vi "Read Firmware and Build Version.vi"(0 "Session Handle in":T1, 11 "error in (no error)":errorcluster) -> (4 "Session Handle out":T1, 6 "Build Date":string, 8 "Firmware Version":string, 15 "error out":errorcluster)   [LabVIEW 2015, in "PAS.lvclass"]
uses:
  PAS.lvclass
  Typedefs/Session Handle.ctl
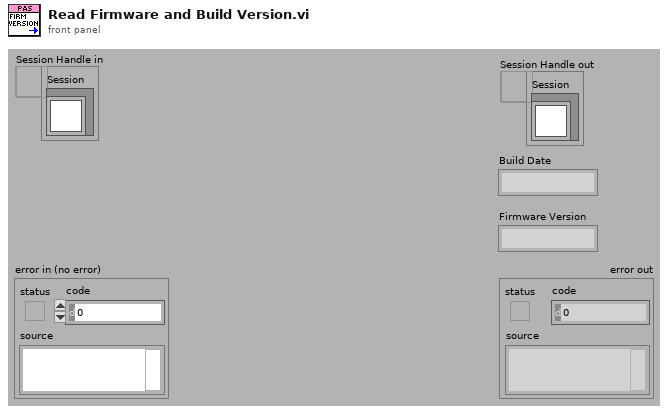
[diagram p1: front panel]
types:
  T1 = typedef "PAS.lvclass/Session Handle.ctl" = refnum<data-value>
  T2 = typedef "XNET Frame CAN.ctl" = cluster{"timestamp":timestamp, "payload":u8[], "identifier":u32, "type":T3, "extended?":bool, "echo?":bool}
  T3 = typedef "XNET Frame Type CAN.ctl" = u8
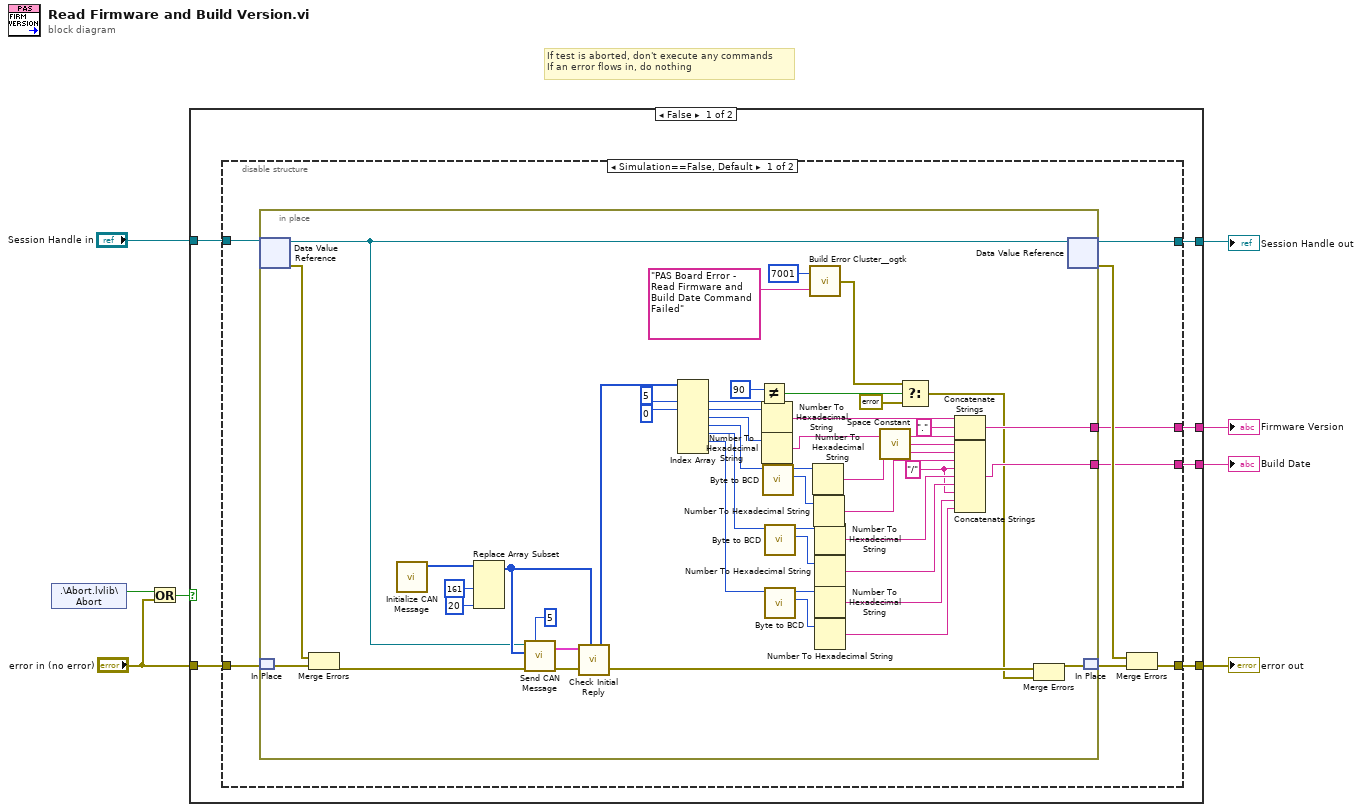
[diagram p0: block diagram]
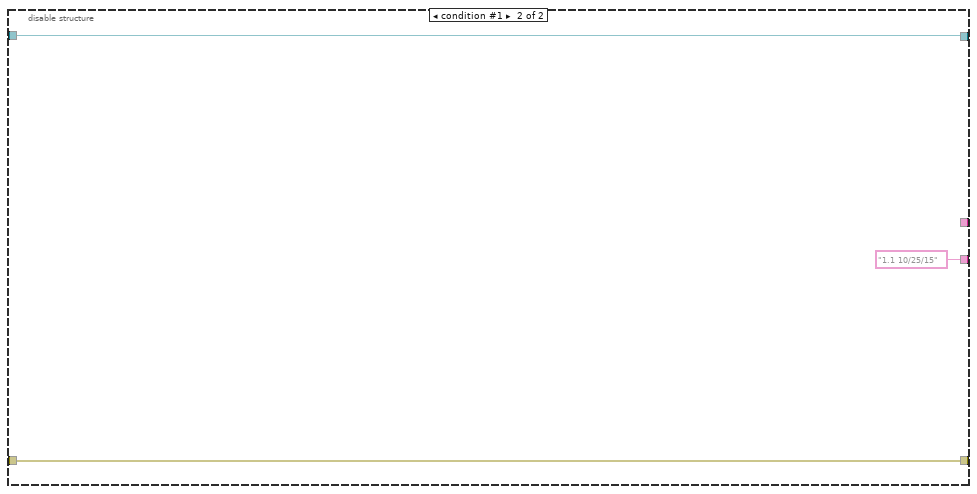
[diagram p2: hidden frame]
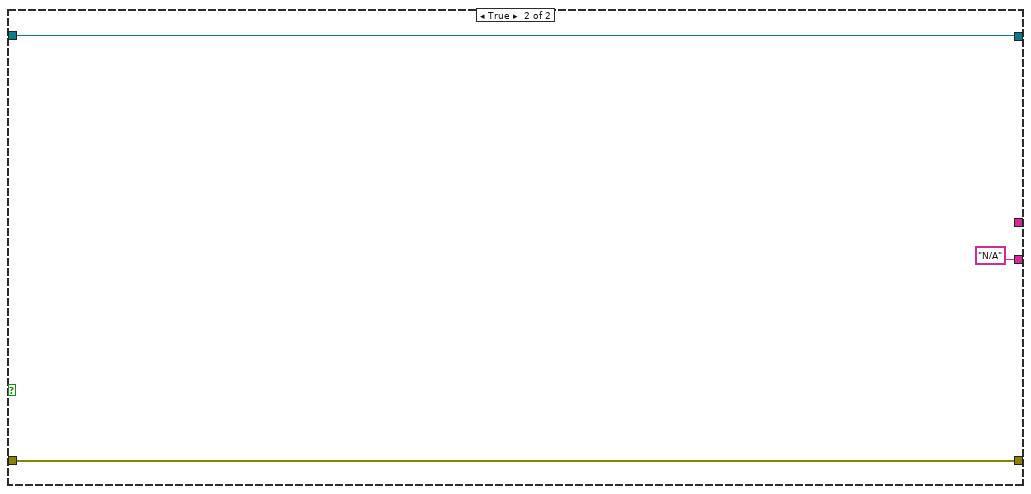
[diagram p3: hidden frame]
diagram:
  # "If test is aborted, don't execute any commands\nIf an error flows in, do nothing"
  n1 = shared-variable ".\\Abort.lvlib\\Abort"() -> (w5:bool)  [unwired: 1 in, 1 out]
  n2 = Or(x=w5, y="error in (no error)") -> (x .or. y?=w3:bool)
  n3 = case shown="False" w3 {
    tunnel: [w14 w75] -> w7
    tunnel: [w13 w74] -> w6
    tunnel: "Session Handle in" -> [w12 w75]
    tunnel: "error in (no error)" -> [w11 w74]
    tunnel: [w10 "N/A"] -> w2
    tunnel: [w9 _] -> w1
    frame False {
      n4 = disable-structure shown="Simulation==False, Default" {
        disable-tunnel: [w22 w72] -> w14
        disable-tunnel: [w19 w71] -> w13
        disable-tunnel: w12 -> [w18 w72]
        disable-tunnel: w11 -> [w17 w71]
        disable-tunnel: [w16 "1.1 10/25/15"] -> w10
        disable-tunnel: [w15 _] -> w9
        frame condition #0 (active) {
          n5 = in-place {
            in-place-border: [w29] -> w16
            in-place-border: [w25] -> w15
            w33 = "/" ("string")
            n6 = in-place-dvr #1(w18) -> (w60:refnum<class "PAS.lvclass">, w64:errorcluster)
            n7 = in-place-match #2(w17) -> (w63:errorcluster)
            n8 = Merge Errors(w64, w63) -> (w62:errorcluster)
            n9 = call "Initialize CAN Message.vi"() -> ("Initial Payload"=w66:u8[])  [unwired: 11 in]
            n10 = Replace Array Subset(array=w66, new element #1=u8 161 ("new element/subarray"), new element #2=u8 20 ("new element/subarray")) -> (w61:u8[])  [unwired: 2 in]
            n11 = call "Send CAN Message.vi"("Number of Retries"=5, "error in (no error)"=w62, "payload"=w61, "Gas In"=w60) -> ("error out"=w24:errorcluster, "Reply"=w58:T2[])  [unwired: 5 in, 1 out]
            n12 = call "Check Initial Reply.vi"("Write Message"=w61, "Reply"=w58) -> ("Data Packet"=w65:u8[])  [unwired: 7 in, 2 out]
            n13 = Index Array(array=w65, index #1=5 ("index"), index #2=0 ("index")) -> (element #1=w52:u8, element #2=w49:u8, element #3=w48:u8, element #4=w47:u8, element #5=w42:u8, element #6=w39:u8)  [unwired: 5 in, 1 out]
            n14 = Not Equal?(x=u8 90 ("new element/subarray"), y=w52) -> (x != y?=w50:bool)
            n15 = Number To Hexadecimal String(2:w49) -> (0:w26:string)  [unwired: 1 in]
            n16 = Number To Hexadecimal String(2:w48) -> (0:w27:string)  [unwired: 1 in]
            n17 = call "Byte to BCD.vi"("U8"=w47) -> ("low nibble"=w45:u8, "hi nibble"=w46:u8)  [unwired: 9 in]
            n18 = call "Byte to BCD.vi"("U8"=w42) -> ("low nibble"=w44:u8, "hi nibble"=w43:u8)  [unwired: 9 in]
            n19 = call "Byte to BCD.vi"("U8"=w39) -> ("low nibble"=w40:u8, "hi nibble"=w41:u8)  [unwired: 9 in]
            n20 = call <userlib>:"Build Error Cluster__ogtk.vi"("String to Prepend to source (\"\")"="PAS Board Error - Read Firmware and Build Date Command Failed" ("string"), "code"=7001) -> ("error out"=w55:errorcluster)
            n21 = Number To Hexadecimal String(2:w46) -> (0:w37:string)  [unwired: 1 in]
            n22 = Number To Hexadecimal String(2:w45) -> (0:w36:string)  [unwired: 1 in]
            n23 = Number To Hexadecimal String(2:w43) -> (0:w35:string)  [unwired: 1 in]
            n24 = Number To Hexadecimal String(2:w44) -> (0:w34:string)  [unwired: 1 in]
            n25 = Number To Hexadecimal String(2:w41) -> (0:w32:string)  [unwired: 1 in]
            n26 = Number To Hexadecimal String(2:w40) -> (0:w31:string)  [unwired: 1 in]
            n27 = call <vilib>:"Space Constant.vi"() -> ("String"=w30:string)
            n28 = Select(t=w55, s=w50, f=errorcluster {"status"=FALSE, "code"=0, "source"=""}) -> (s? t:f=w23:errorcluster)
            n29 = Concatenate Strings(w26, "." ("string"), w27) -> (w25:string)
            n30 = Concatenate Strings(w30, w37, w36, w33, w35, w34, w33, w32, w31) -> (w29:string)
            n31 = Merge Errors(w24, w23) -> (w67:errorcluster)
            n32 = in-place-dvr #1(w60) -> (w22:T1, w20:errorcluster)
            n33 = in-place-match #2(w67) -> (w21:errorcluster)
          }
          n34 = Merge Errors(w20, w21) -> (w19:errorcluster)
        }
        frame condition #1 {
        }
      }
    }
    frame True {
    }
  }
  "Session Handle out" <- w7
  "error out" <- w6
  "Build Date" <- w2
  "Firmware Version" <- w1
